vi "manual_valve_testing.vi"() -> ()   [LabVIEW 2022 SP3]
uses:
  <vilib>/Instr/_visa.llb/VISA Configure Serial Port (Instr).vi
panel:
  out "error out 4":errorcluster
  out "error out 3":errorcluster
  out "error out 2":errorcluster
  out "error out":errorcluster
  in  "?":bool
  in  "?":bool
  in  "?":bool
  in  "?":bool
  in  "?":bool
  in  "?":bool
  in  "?":bool
  in  "?":bool
  in  "?":bool
  in  "?":bool
  in  "?":bool
  in  "?":bool
  in  "?":bool
  in  "?":bool
  in  "?":bool
  in  "?":bool
  in  "?":bool
  in  "?":bool
  in  "?":bool
  in  "?":bool
  in  "?":bool
  in  "?":bool
  in  "?":bool
  in  "?":bool
  in  "?":bool
  in  "?":bool
  in  "?":bool
  in  "?":bool
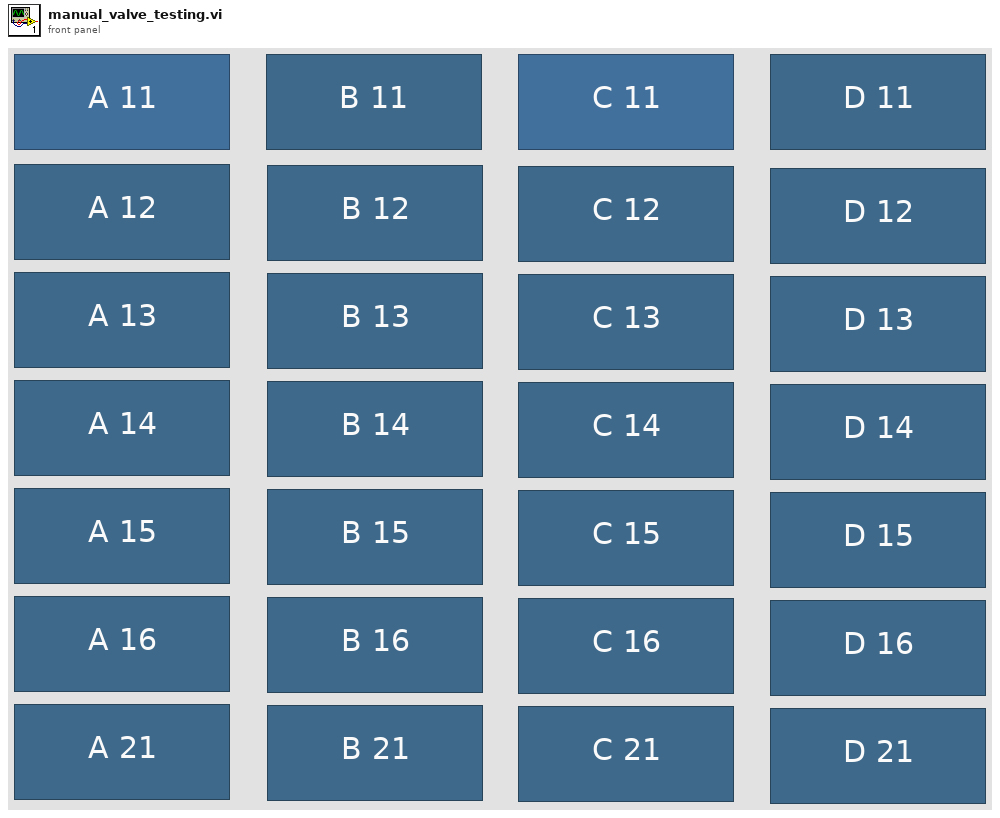
[diagram p1: front panel]
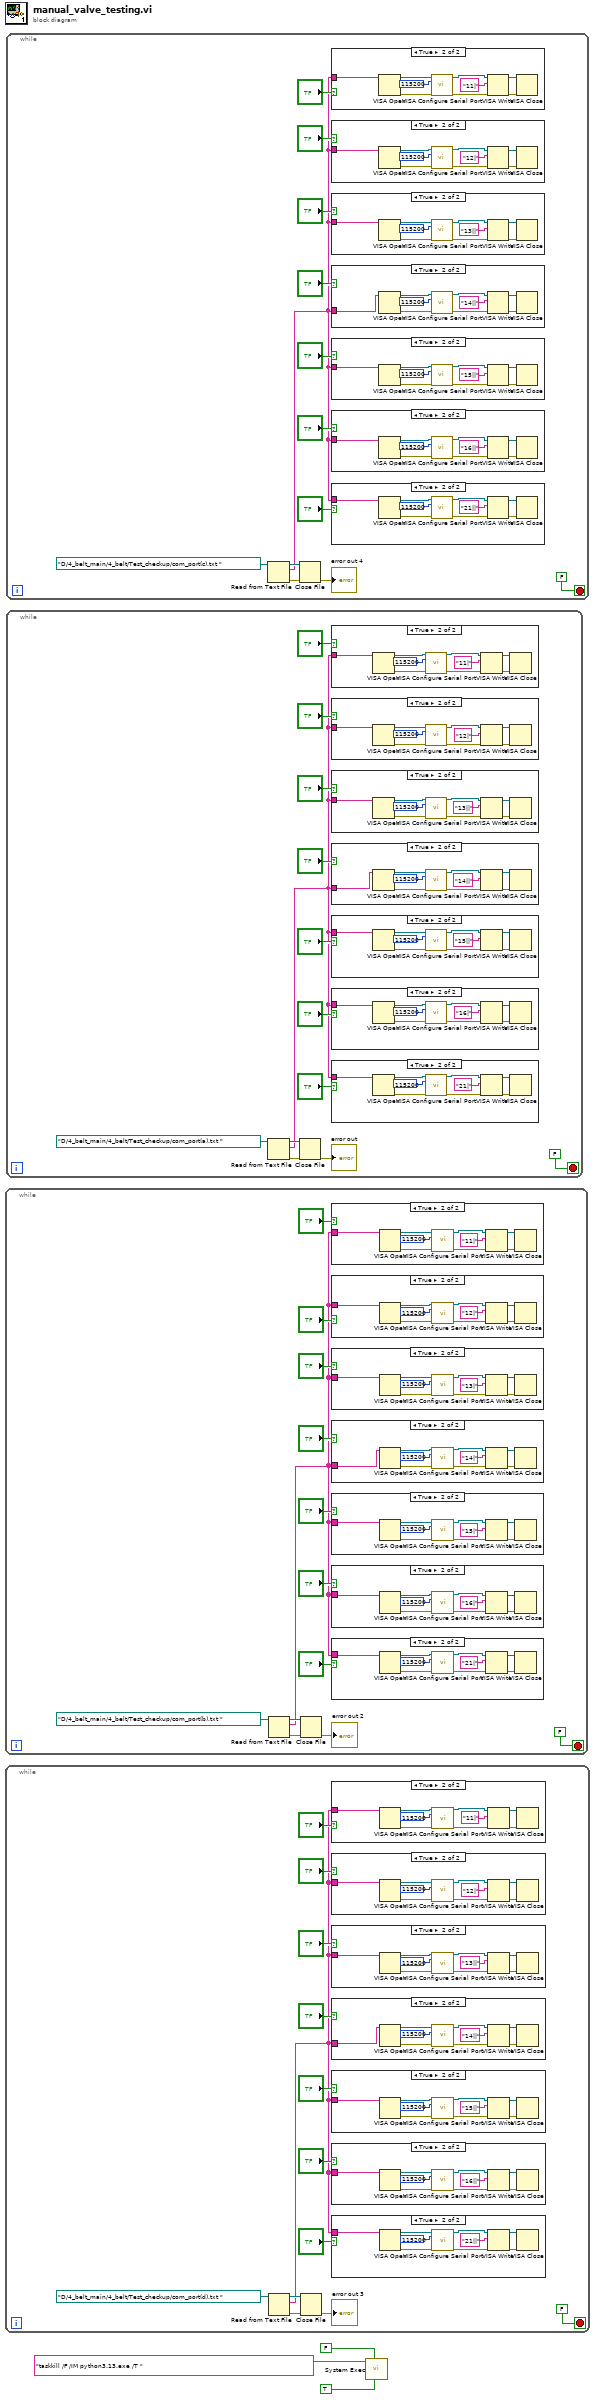
[diagram p0: block diagram]
diagram:
  n1 = while {
    stop <- FALSE stop-if-true
    n2 = Read from Text File(file (use dialog)=path "D:/4_belt_main/4_belt/Test_checkup/com_port(b).txt ") -> (refnum out=w6:refnum<file>, text=w4:string, error out=w7:errorcluster)  [unwired: 3 in, 1 out]
    n3 = Close File(refnum=w6, error in=w7) -> (error out=→"error out 2":errorcluster)  [unwired: 1 out]
    n4 = case shown="True" "?" {
      tunnel: w4 -> [_ w64]
      frame False {
      }
      frame True {
        n5 = VISA Open(VISA resource name=w64) -> (VISA resource name=w65:refnum<visa-resource-name>, error out=w68:errorcluster)  [unwired: 4 in]
        n6 = call-poly "VISA Configure Serial Port"("VISA resource name"=w65, "baud rate (9600)"=u32 115200, "error in (no error)"=w68) -> ("VISA resource name out"=w66:refnum<visa-resource-name>, "error out"=w69:errorcluster)  [unwired: 11 in]
        n7 = VISA Write(VISA resource name=w66, write buffer="11|", error in (no error)=w69) -> (VISA resource name out=w70:refnum<visa-resource-name>, error out=w67:errorcluster)  [unwired: 1 out]
        n8 = VISA Close(VISA resource name=w70, error in (no error)=w67) -> ()  [unwired: 1 out]
      }
    }
    n9 = case shown="True" "?" {
      tunnel: w4 -> [_ w55]
      frame False {
      }
      frame True {
        n10 = VISA Open(VISA resource name=w55) -> (VISA resource name=w56:refnum<visa-resource-name>, error out=w59:errorcluster)  [unwired: 4 in]
        n11 = call-poly "VISA Configure Serial Port"("VISA resource name"=w56, "baud rate (9600)"=u32 115200, "error in (no error)"=w59) -> ("VISA resource name out"=w57:refnum<visa-resource-name>, "error out"=w60:errorcluster)  [unwired: 11 in]
        n12 = VISA Write(VISA resource name=w57, write buffer="12|", error in (no error)=w60) -> (VISA resource name out=w61:refnum<visa-resource-name>, error out=w58:errorcluster)  [unwired: 1 out]
        n13 = VISA Close(VISA resource name=w61, error in (no error)=w58) -> ()  [unwired: 1 out]
      }
    }
    n14 = case shown="True" "?" {
      tunnel: w4 -> [_ w73]
      frame False {
      }
      frame True {
        n15 = VISA Open(VISA resource name=w73) -> (VISA resource name=w74:refnum<visa-resource-name>, error out=w77:errorcluster)  [unwired: 4 in]
        n16 = call-poly "VISA Configure Serial Port"("VISA resource name"=w74, "baud rate (9600)"=u32 115200, "error in (no error)"=w77) -> ("VISA resource name out"=w75:refnum<visa-resource-name>, "error out"=w78:errorcluster)  [unwired: 11 in]
        n17 = VISA Write(VISA resource name=w75, write buffer="13|", error in (no error)=w78) -> (VISA resource name out=w79:refnum<visa-resource-name>, error out=w76:errorcluster)  [unwired: 1 out]
        n18 = VISA Close(VISA resource name=w79, error in (no error)=w76) -> ()  [unwired: 1 out]
      }
    }
    n19 = case shown="True" "?" {
      tunnel: w4 -> [_ w44]
      frame False {
      }
      frame True {
        n20 = VISA Open(VISA resource name=w44) -> (VISA resource name=w47:refnum<visa-resource-name>, error out=w50:errorcluster)  [unwired: 4 in]
        n21 = call-poly "VISA Configure Serial Port"("VISA resource name"=w47, "baud rate (9600)"=u32 115200, "error in (no error)"=w50) -> ("VISA resource name out"=w48:refnum<visa-resource-name>, "error out"=w51:errorcluster)  [unwired: 11 in]
        n22 = VISA Write(VISA resource name=w48, write buffer="14|", error in (no error)=w51) -> (VISA resource name out=w52:refnum<visa-resource-name>, error out=w49:errorcluster)  [unwired: 1 out]
        n23 = VISA Close(VISA resource name=w52, error in (no error)=w49) -> ()  [unwired: 1 out]
      }
    }
    n24 = case shown="True" "?" {
      tunnel: w4 -> [_ w35]
      frame False {
      }
      frame True {
        n25 = VISA Open(VISA resource name=w35) -> (VISA resource name=w38:refnum<visa-resource-name>, error out=w41:errorcluster)  [unwired: 4 in]
        n26 = call-poly "VISA Configure Serial Port"("VISA resource name"=w38, "baud rate (9600)"=u32 115200, "error in (no error)"=w41) -> ("VISA resource name out"=w39:refnum<visa-resource-name>, "error out"=w42:errorcluster)  [unwired: 11 in]
        n27 = VISA Write(VISA resource name=w39, write buffer="15|", error in (no error)=w42) -> (VISA resource name out=w43:refnum<visa-resource-name>, error out=w40:errorcluster)  [unwired: 1 out]
        n28 = VISA Close(VISA resource name=w43, error in (no error)=w40) -> ()  [unwired: 1 out]
      }
    }
    n29 = case shown="True" "?" {
      tunnel: w4 -> [_ w26]
      frame False {
      }
      frame True {
        n30 = VISA Open(VISA resource name=w26) -> (VISA resource name=w29:refnum<visa-resource-name>, error out=w32:errorcluster)  [unwired: 4 in]
        n31 = call-poly "VISA Configure Serial Port"("VISA resource name"=w29, "baud rate (9600)"=u32 115200, "error in (no error)"=w32) -> ("VISA resource name out"=w30:refnum<visa-resource-name>, "error out"=w33:errorcluster)  [unwired: 11 in]
        n32 = VISA Write(VISA resource name=w30, write buffer="16|", error in (no error)=w33) -> (VISA resource name out=w34:refnum<visa-resource-name>, error out=w31:errorcluster)  [unwired: 1 out]
        n33 = VISA Close(VISA resource name=w34, error in (no error)=w31) -> ()  [unwired: 1 out]
      }
    }
    n34 = case shown="True" "?" {
      tunnel: w4 -> [_ w17]
      frame False {
      }
      frame True {
        n35 = VISA Open(VISA resource name=w17) -> (VISA resource name=w20:refnum<visa-resource-name>, error out=w23:errorcluster)  [unwired: 4 in]
        n36 = call-poly "VISA Configure Serial Port"("VISA resource name"=w20, "baud rate (9600)"=u32 115200, "error in (no error)"=w23) -> ("VISA resource name out"=w21:refnum<visa-resource-name>, "error out"=w24:errorcluster)  [unwired: 11 in]
        n37 = VISA Write(VISA resource name=w21, write buffer="21|", error in (no error)=w24) -> (VISA resource name out=w25:refnum<visa-resource-name>, error out=w22:errorcluster)  [unwired: 1 out]
        n38 = VISA Close(VISA resource name=w25, error in (no error)=w22) -> ()  [unwired: 1 out]
      }
    }
  }
  n39 = while {
    stop <- FALSE stop-if-true
    n40 = Read from Text File(file (use dialog)=path "D:/4_belt_main/4_belt/Test_checkup/com_port(d).txt ") -> (refnum out=w82:refnum<file>, text=w80:string, error out=w83:errorcluster)  [unwired: 3 in, 1 out]
    n41 = Close File(refnum=w82, error in=w83) -> (error out=→"error out 3":errorcluster)  [unwired: 1 out]
    n42 = case shown="True" "?" {
      tunnel: w80 -> [_ w140]
      frame False {
      }
      frame True {
        n43 = VISA Open(VISA resource name=w140) -> (VISA resource name=w141:refnum<visa-resource-name>, error out=w144:errorcluster)  [unwired: 4 in]
        n44 = call-poly "VISA Configure Serial Port"("VISA resource name"=w141, "baud rate (9600)"=u32 115200, "error in (no error)"=w144) -> ("VISA resource name out"=w142:refnum<visa-resource-name>, "error out"=w145:errorcluster)  [unwired: 11 in]
        n45 = VISA Write(VISA resource name=w142, write buffer="11|", error in (no error)=w145) -> (VISA resource name out=w146:refnum<visa-resource-name>, error out=w143:errorcluster)  [unwired: 1 out]
        n46 = VISA Close(VISA resource name=w146, error in (no error)=w143) -> ()  [unwired: 1 out]
      }
    }
    n47 = case shown="True" "?" {
      tunnel: w80 -> [_ w131]
      frame False {
      }
      frame True {
        n48 = VISA Open(VISA resource name=w131) -> (VISA resource name=w132:refnum<visa-resource-name>, error out=w135:errorcluster)  [unwired: 4 in]
        n49 = call-poly "VISA Configure Serial Port"("VISA resource name"=w132, "baud rate (9600)"=u32 115200, "error in (no error)"=w135) -> ("VISA resource name out"=w133:refnum<visa-resource-name>, "error out"=w136:errorcluster)  [unwired: 11 in]
        n50 = VISA Write(VISA resource name=w133, write buffer="12|", error in (no error)=w136) -> (VISA resource name out=w137:refnum<visa-resource-name>, error out=w134:errorcluster)  [unwired: 1 out]
        n51 = VISA Close(VISA resource name=w137, error in (no error)=w134) -> ()  [unwired: 1 out]
      }
    }
    n52 = case shown="True" "?" {
      tunnel: w80 -> [_ w149]
      frame False {
      }
      frame True {
        n53 = VISA Open(VISA resource name=w149) -> (VISA resource name=w150:refnum<visa-resource-name>, error out=w153:errorcluster)  [unwired: 4 in]
        n54 = call-poly "VISA Configure Serial Port"("VISA resource name"=w150, "baud rate (9600)"=u32 115200, "error in (no error)"=w153) -> ("VISA resource name out"=w151:refnum<visa-resource-name>, "error out"=w154:errorcluster)  [unwired: 11 in]
        n55 = VISA Write(VISA resource name=w151, write buffer="13||", error in (no error)=w154) -> (VISA resource name out=w155:refnum<visa-resource-name>, error out=w152:errorcluster)  [unwired: 1 out]
        n56 = VISA Close(VISA resource name=w155, error in (no error)=w152) -> ()  [unwired: 1 out]
      }
    }
    n57 = case shown="True" "?" {
      tunnel: w80 -> [_ w120]
      frame False {
      }
      frame True {
        n58 = VISA Open(VISA resource name=w120) -> (VISA resource name=w123:refnum<visa-resource-name>, error out=w126:errorcluster)  [unwired: 4 in]
        n59 = call-poly "VISA Configure Serial Port"("VISA resource name"=w123, "baud rate (9600)"=u32 115200, "error in (no error)"=w126) -> ("VISA resource name out"=w124:refnum<visa-resource-name>, "error out"=w127:errorcluster)  [unwired: 11 in]
        n60 = VISA Write(VISA resource name=w124, write buffer="14||", error in (no error)=w127) -> (VISA resource name out=w128:refnum<visa-resource-name>, error out=w125:errorcluster)  [unwired: 1 out]
        n61 = VISA Close(VISA resource name=w128, error in (no error)=w125) -> ()  [unwired: 1 out]
      }
    }
    n62 = case shown="True" "?" {
      tunnel: w80 -> [_ w111]
      frame False {
      }
      frame True {
        n63 = VISA Open(VISA resource name=w111) -> (VISA resource name=w114:refnum<visa-resource-name>, error out=w117:errorcluster)  [unwired: 4 in]
        n64 = call-poly "VISA Configure Serial Port"("VISA resource name"=w114, "baud rate (9600)"=u32 115200, "error in (no error)"=w117) -> ("VISA resource name out"=w115:refnum<visa-resource-name>, "error out"=w118:errorcluster)  [unwired: 11 in]
        n65 = VISA Write(VISA resource name=w115, write buffer="15||", error in (no error)=w118) -> (VISA resource name out=w119:refnum<visa-resource-name>, error out=w116:errorcluster)  [unwired: 1 out]
        n66 = VISA Close(VISA resource name=w119, error in (no error)=w116) -> ()  [unwired: 1 out]
      }
    }
    n67 = case shown="True" "?" {
      tunnel: w80 -> [_ w102]
      frame False {
      }
      frame True {
        n68 = VISA Open(VISA resource name=w102) -> (VISA resource name=w105:refnum<visa-resource-name>, error out=w108:errorcluster)  [unwired: 4 in]
        n69 = call-poly "VISA Configure Serial Port"("VISA resource name"=w105, "baud rate (9600)"=u32 115200, "error in (no error)"=w108) -> ("VISA resource name out"=w106:refnum<visa-resource-name>, "error out"=w109:errorcluster)  [unwired: 11 in]
        n70 = VISA Write(VISA resource name=w106, write buffer="16||", error in (no error)=w109) -> (VISA resource name out=w110:refnum<visa-resource-name>, error out=w107:errorcluster)  [unwired: 1 out]
        n71 = VISA Close(VISA resource name=w110, error in (no error)=w107) -> ()  [unwired: 1 out]
      }
    }
    n72 = case shown="True" "?" {
      tunnel: w80 -> [_ w93]
      frame False {
      }
      frame True {
        n73 = VISA Open(VISA resource name=w93) -> (VISA resource name=w96:refnum<visa-resource-name>, error out=w99:errorcluster)  [unwired: 4 in]
        n74 = call-poly "VISA Configure Serial Port"("VISA resource name"=w96, "baud rate (9600)"=u32 115200, "error in (no error)"=w99) -> ("VISA resource name out"=w97:refnum<visa-resource-name>, "error out"=w100:errorcluster)  [unwired: 11 in]
        n75 = VISA Write(VISA resource name=w97, write buffer="21||", error in (no error)=w100) -> (VISA resource name out=w101:refnum<visa-resource-name>, error out=w98:errorcluster)  [unwired: 1 out]
        n76 = VISA Close(VISA resource name=w101, error in (no error)=w98) -> ()  [unwired: 1 out]
      }
    }
  }
  n77 = while {
    stop <- FALSE stop-if-true
    n78 = Read from Text File(file (use dialog)=path "D:/4_belt_main/4_belt/Test_checkup/com_port(a).txt ") -> (refnum out=w158:refnum<file>, text=w156:string, error out=w159:errorcluster)  [unwired: 3 in, 1 out]
    n79 = Close File(refnum=w158, error in=w159) -> (error out=→"error out":errorcluster)  [unwired: 1 out]
    n80 = case shown="True" "?" {
      tunnel: w156 -> [_ w216]
      frame False {
      }
      frame True {
        n81 = VISA Open(VISA resource name=w216) -> (VISA resource name=w217:refnum<visa-resource-name>, error out=w220:errorcluster)  [unwired: 4 in]
        n82 = call-poly "VISA Configure Serial Port"("VISA resource name"=w217, "baud rate (9600)"=u32 115200, "error in (no error)"=w220) -> ("VISA resource name out"=w218:refnum<visa-resource-name>, "error out"=w221:errorcluster)  [unwired: 11 in]
        n83 = VISA Write(VISA resource name=w218, write buffer="11|", error in (no error)=w221) -> (VISA resource name out=w222:refnum<visa-resource-name>, error out=w219:errorcluster)  [unwired: 1 out]
        n84 = VISA Close(VISA resource name=w222, error in (no error)=w219) -> ()  [unwired: 1 out]
      }
    }
    n85 = case shown="True" "?" {
      tunnel: w156 -> [_ w207]
      frame False {
      }
      frame True {
        n86 = VISA Open(VISA resource name=w207) -> (VISA resource name=w208:refnum<visa-resource-name>, error out=w211:errorcluster)  [unwired: 4 in]
        n87 = call-poly "VISA Configure Serial Port"("VISA resource name"=w208, "baud rate (9600)"=u32 115200, "error in (no error)"=w211) -> ("VISA resource name out"=w209:refnum<visa-resource-name>, "error out"=w212:errorcluster)  [unwired: 11 in]
        n88 = VISA Write(VISA resource name=w209, write buffer="12|", error in (no error)=w212) -> (VISA resource name out=w213:refnum<visa-resource-name>, error out=w210:errorcluster)  [unwired: 1 out]
        n89 = VISA Close(VISA resource name=w213, error in (no error)=w210) -> ()  [unwired: 1 out]
      }
    }
    n90 = case shown="True" "?" {
      tunnel: w156 -> [_ w225]
      frame False {
      }
      frame True {
        n91 = VISA Open(VISA resource name=w225) -> (VISA resource name=w226:refnum<visa-resource-name>, error out=w229:errorcluster)  [unwired: 4 in]
        n92 = call-poly "VISA Configure Serial Port"("VISA resource name"=w226, "baud rate (9600)"=u32 115200, "error in (no error)"=w229) -> ("VISA resource name out"=w227:refnum<visa-resource-name>, "error out"=w230:errorcluster)  [unwired: 11 in]
        n93 = VISA Write(VISA resource name=w227, write buffer="13||", error in (no error)=w230) -> (VISA resource name out=w231:refnum<visa-resource-name>, error out=w228:errorcluster)  [unwired: 1 out]
        n94 = VISA Close(VISA resource name=w231, error in (no error)=w228) -> ()  [unwired: 1 out]
      }
    }
    n95 = case shown="True" "?" {
      tunnel: w156 -> [_ w196]
      frame False {
      }
      frame True {
        n96 = VISA Open(VISA resource name=w196) -> (VISA resource name=w199:refnum<visa-resource-name>, error out=w202:errorcluster)  [unwired: 4 in]
        n97 = call-poly "VISA Configure Serial Port"("VISA resource name"=w199, "baud rate (9600)"=u32 115200, "error in (no error)"=w202) -> ("VISA resource name out"=w200:refnum<visa-resource-name>, "error out"=w203:errorcluster)  [unwired: 11 in]
        n98 = VISA Write(VISA resource name=w200, write buffer="14||", error in (no error)=w203) -> (VISA resource name out=w204:refnum<visa-resource-name>, error out=w201:errorcluster)  [unwired: 1 out]
        n99 = VISA Close(VISA resource name=w204, error in (no error)=w201) -> ()  [unwired: 1 out]
      }
    }
    n100 = case shown="True" "?" {
      tunnel: w156 -> [_ w187]
      frame False {
      }
      frame True {
        n101 = VISA Open(VISA resource name=w187) -> (VISA resource name=w190:refnum<visa-resource-name>, error out=w193:errorcluster)  [unwired: 4 in]
        n102 = call-poly "VISA Configure Serial Port"("VISA resource name"=w190, "baud rate (9600)"=u32 115200, "error in (no error)"=w193) -> ("VISA resource name out"=w191:refnum<visa-resource-name>, "error out"=w194:errorcluster)  [unwired: 11 in]
        n103 = VISA Write(VISA resource name=w191, write buffer="15||", error in (no error)=w194) -> (VISA resource name out=w195:refnum<visa-resource-name>, error out=w192:errorcluster)  [unwired: 1 out]
        n104 = VISA Close(VISA resource name=w195, error in (no error)=w192) -> ()  [unwired: 1 out]
      }
    }
    n105 = case shown="True" "?" {
      tunnel: w156 -> [_ w178]
      frame False {
      }
      frame True {
        n106 = VISA Open(VISA resource name=w178) -> (VISA resource name=w181:refnum<visa-resource-name>, error out=w184:errorcluster)  [unwired: 4 in]
        n107 = call-poly "VISA Configure Serial Port"("VISA resource name"=w181, "baud rate (9600)"=u32 115200, "error in (no error)"=w184) -> ("VISA resource name out"=w182:refnum<visa-resource-name>, "error out"=w185:errorcluster)  [unwired: 11 in]
        n108 = VISA Write(VISA resource name=w182, write buffer="16|", error in (no error)=w185) -> (VISA resource name out=w186:refnum<visa-resource-name>, error out=w183:errorcluster)  [unwired: 1 out]
        n109 = VISA Close(VISA resource name=w186, error in (no error)=w183) -> ()  [unwired: 1 out]
      }
    }
    n110 = case shown="True" "?" {
      tunnel: w156 -> [_ w169]
      frame False {
      }
      frame True {
        n111 = VISA Open(VISA resource name=w169) -> (VISA resource name=w172:refnum<visa-resource-name>, error out=w175:errorcluster)  [unwired: 4 in]
        n112 = call-poly "VISA Configure Serial Port"("VISA resource name"=w172, "baud rate (9600)"=u32 115200, "error in (no error)"=w175) -> ("VISA resource name out"=w173:refnum<visa-resource-name>, "error out"=w176:errorcluster)  [unwired: 11 in]
        n113 = VISA Write(VISA resource name=w173, write buffer="21|", error in (no error)=w176) -> (VISA resource name out=w177:refnum<visa-resource-name>, error out=w174:errorcluster)  [unwired: 1 out]
        n114 = VISA Close(VISA resource name=w177, error in (no error)=w174) -> ()  [unwired: 1 out]
      }
    }
  }
  n115 = while {
    stop <- FALSE stop-if-true
    n116 = Read from Text File(file (use dialog)=path "D:/4_belt_main/4_belt/Test_checkup/com_port(c).txt ") -> (refnum out=w234:refnum<file>, text=w232:string, error out=w235:errorcluster)  [unwired: 3 in, 1 out]
    n117 = Close File(refnum=w234, error in=w235) -> (error out=→"error out 4":errorcluster)  [unwired: 1 out]
    n118 = case shown="True" "?" {
      tunnel: w232 -> [_ w292]
      frame False {
      }
      frame True {
        n119 = VISA Open(VISA resource name=w292) -> (VISA resource name=w293:refnum<visa-resource-name>, error out=w296:errorcluster)  [unwired: 4 in]
        n120 = call-poly "VISA Configure Serial Port"("VISA resource name"=w293, "baud rate (9600)"=u32 115200, "error in (no error)"=w296) -> ("VISA resource name out"=w294:refnum<visa-resource-name>, "error out"=w297:errorcluster)  [unwired: 11 in]
        n121 = VISA Write(VISA resource name=w294, write buffer="11|", error in (no error)=w297) -> (VISA resource name out=w298:refnum<visa-resource-name>, error out=w295:errorcluster)  [unwired: 1 out]
        n122 = VISA Close(VISA resource name=w298, error in (no error)=w295) -> ()  [unwired: 1 out]
      }
    }
    n123 = case shown="True" "?" {
      tunnel: w232 -> [_ w283]
      frame False {
      }
      frame True {
        n124 = VISA Open(VISA resource name=w283) -> (VISA resource name=w284:refnum<visa-resource-name>, error out=w287:errorcluster)  [unwired: 4 in]
        n125 = call-poly "VISA Configure Serial Port"("VISA resource name"=w284, "baud rate (9600)"=u32 115200, "error in (no error)"=w287) -> ("VISA resource name out"=w285:refnum<visa-resource-name>, "error out"=w288:errorcluster)  [unwired: 11 in]
        n126 = VISA Write(VISA resource name=w285, write buffer="12|", error in (no error)=w288) -> (VISA resource name out=w289:refnum<visa-resource-name>, error out=w286:errorcluster)  [unwired: 1 out]
        n127 = VISA Close(VISA resource name=w289, error in (no error)=w286) -> ()  [unwired: 1 out]
      }
    }
    n128 = case shown="True" "?" {
      tunnel: w232 -> [_ w301]
      frame False {
      }
      frame True {
        n129 = VISA Open(VISA resource name=w301) -> (VISA resource name=w302:refnum<visa-resource-name>, error out=w305:errorcluster)  [unwired: 4 in]
        n130 = call-poly "VISA Configure Serial Port"("VISA resource name"=w302, "baud rate (9600)"=u32 115200, "error in (no error)"=w305) -> ("VISA resource name out"=w303:refnum<visa-resource-name>, "error out"=w306:errorcluster)  [unwired: 11 in]
        n131 = VISA Write(VISA resource name=w303, write buffer="13||", error in (no error)=w306) -> (VISA resource name out=w307:refnum<visa-resource-name>, error out=w304:errorcluster)  [unwired: 1 out]
        n132 = VISA Close(VISA resource name=w307, error in (no error)=w304) -> ()  [unwired: 1 out]
      }
    }
    n133 = case shown="True" "?" {
      tunnel: w232 -> [_ w272]
      frame False {
      }
      frame True {
        n134 = VISA Open(VISA resource name=w272) -> (VISA resource name=w275:refnum<visa-resource-name>, error out=w278:errorcluster)  [unwired: 4 in]
        n135 = call-poly "VISA Configure Serial Port"("VISA resource name"=w275, "baud rate (9600)"=u32 115200, "error in (no error)"=w278) -> ("VISA resource name out"=w276:refnum<visa-resource-name>, "error out"=w279:errorcluster)  [unwired: 11 in]
        n136 = VISA Write(VISA resource name=w276, write buffer="14||", error in (no error)=w279) -> (VISA resource name out=w280:refnum<visa-resource-name>, error out=w277:errorcluster)  [unwired: 1 out]
        n137 = VISA Close(VISA resource name=w280, error in (no error)=w277) -> ()  [unwired: 1 out]
      }
    }
    n138 = case shown="True" "?" {
      tunnel: w232 -> [_ w263]
      frame False {
      }
      frame True {
        n139 = VISA Open(VISA resource name=w263) -> (VISA resource name=w266:refnum<visa-resource-name>, error out=w269:errorcluster)  [unwired: 4 in]
        n140 = call-poly "VISA Configure Serial Port"("VISA resource name"=w266, "baud rate (9600)"=u32 115200, "error in (no error)"=w269) -> ("VISA resource name out"=w267:refnum<visa-resource-name>, "error out"=w270:errorcluster)  [unwired: 11 in]
        n141 = VISA Write(VISA resource name=w267, write buffer="15||", error in (no error)=w270) -> (VISA resource name out=w271:refnum<visa-resource-name>, error out=w268:errorcluster)  [unwired: 1 out]
        n142 = VISA Close(VISA resource name=w271, error in (no error)=w268) -> ()  [unwired: 1 out]
      }
    }
    n143 = case shown="True" "?" {
      tunnel: w232 -> [_ w254]
      frame False {
      }
      frame True {
        n144 = VISA Open(VISA resource name=w254) -> (VISA resource name=w257:refnum<visa-resource-name>, error out=w260:errorcluster)  [unwired: 4 in]
        n145 = call-poly "VISA Configure Serial Port"("VISA resource name"=w257, "baud rate (9600)"=u32 115200, "error in (no error)"=w260) -> ("VISA resource name out"=w258:refnum<visa-resource-name>, "error out"=w261:errorcluster)  [unwired: 11 in]
        n146 = VISA Write(VISA resource name=w258, write buffer="16||", error in (no error)=w261) -> (VISA resource name out=w262:refnum<visa-resource-name>, error out=w259:errorcluster)  [unwired: 1 out]
        n147 = VISA Close(VISA resource name=w262, error in (no error)=w259) -> ()  [unwired: 1 out]
      }
    }
    n148 = case shown="True" "?" {
      tunnel: w232 -> [_ w245]
      frame False {
      }
      frame True {
        n149 = VISA Open(VISA resource name=w245) -> (VISA resource name=w248:refnum<visa-resource-name>, error out=w251:errorcluster)  [unwired: 4 in]
        n150 = call-poly "VISA Configure Serial Port"("VISA resource name"=w248, "baud rate (9600)"=u32 115200, "error in (no error)"=w251) -> ("VISA resource name out"=w249:refnum<visa-resource-name>, "error out"=w252:errorcluster)  [unwired: 11 in]
        n151 = VISA Write(VISA resource name=w249, write buffer="21||", error in (no error)=w252) -> (VISA resource name out=w253:refnum<visa-resource-name>, error out=w250:errorcluster)  [unwired: 1 out]
        n152 = VISA Close(VISA resource name=w253, error in (no error)=w250) -> ()  [unwired: 1 out]
      }
    }
  }
  n153 = call <vilib>:"System Exec.vi"("run minimized? (F)"=TRUE, "wait until completion? (T)"=FALSE, "command line"="taskkill /F /IM python3.13.exe /T ") -> ()  [unwired: 5 in, 4 out]
